vi "函数类型1测试 - 副本 (3).vi"() -> ()   [LabVIEW 2010]
panel:
  out "light_32":bool
  out "light_31":bool
  out "light_30":bool
  out "light_29":bool
  out "light_28":bool
  out "light_27":bool
  out "light_26":bool
  out "light_25":bool
  out "light_24":bool
  out "light_23":bool
  out "light_22":bool
  out "light_21":bool
  out "light_20":bool
  out "light_19":bool
  out "light_18":bool
  out "light_17":bool
  out "light_16":bool
  out "light_15":bool
  out "light_14":bool
  out "light_13":bool
  out "light_12":bool
  out "light_11":bool
  out "light_10":bool
  out "light_9":bool
  out "light_8":bool
  out "light_7":bool
  out "light_6":bool
  out "light_5":bool
  out "light_4":bool
  out "light_3":bool
  out "light_2":bool
  out "light_1":bool
  in  "A_16":bool
  in  "A_15":bool
  in  "A_14":bool
  in  "A_13":bool
  in  "A_12":bool
  in  "A_11":bool
  in  "A_10":bool
  in  "A_9":bool
  in  "A_8":bool
  in  "A_7":bool
  in  "A_6":bool
  in  "A_5":bool
  in  "A_4":bool
  in  "A_3":bool
  in  "A_2":bool
  in  "A_1":bool
  out "temp":string
  out "bstart":bool
  in  "同步_1":i32
  in  "数组_反馈值":dbl[][](array[numeric])
  in  "第几个数据":i32
  in  "第几组数据":i32
  out "Analog_WC":string[][](table) caption="表格"
  in  "数组_设定值":dbl[][](array[numeric])
  in  "数组_选择":bool[](array[boolean])
  out "Analog_back":string[][](table) caption="表格"
  in  "A_32":bool
  in  "A_31":bool
  in  "A_30":bool
  in  "A_29":bool
  in  "A_28":bool
  in  "A_27":bool
  in  "A_26":bool
  in  "A_25":bool
  in  "A_24":bool
  in  "A_23":bool
  in  "A_22":bool
  in  "A_21":bool
  in  "A_20":bool
  in  "A_19":bool
  in  "A_18":bool
  in  "A_17":bool
  in  "Analog_IN":string[][](table) caption="表格"
  out "退出？":bool
  out "合格？":bool[][](array[boolean])
  out "测试结论":string
  in  "btn_反选":bool
  in  "btn_全选":bool
  in  "btn_开始测试":bool
  in  "btn_取消":bool
  # "模拟量选择及输入值（V）"
  # "模拟量反馈值（V）"
  # "模拟量误差值（%）"
  # "从0开始"
  # "从1开始,第0列没有使用"
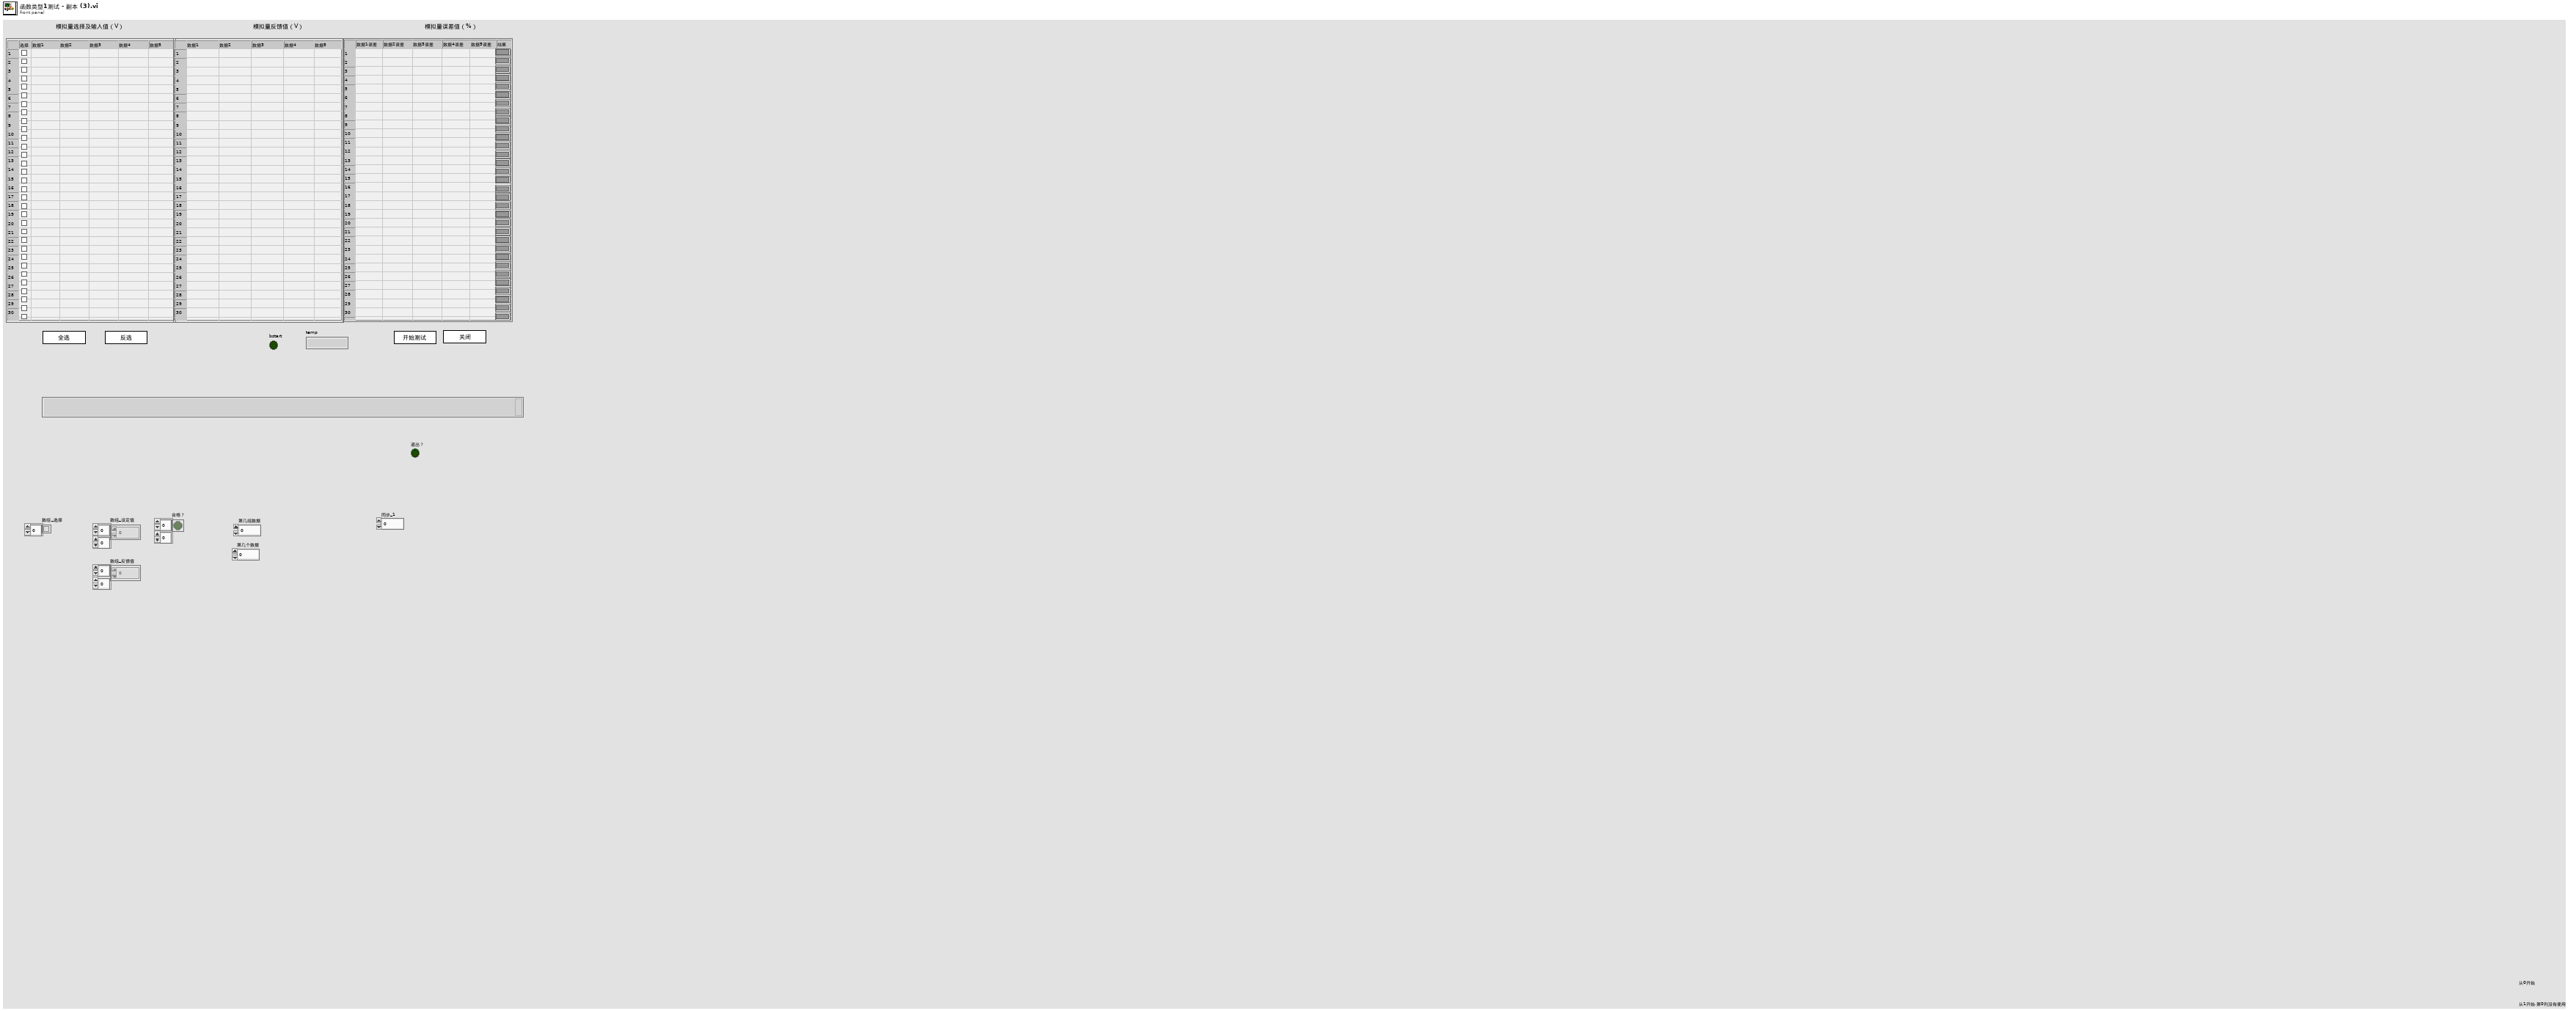
[diagram p1: front panel]
types:
  T1 = enum8{"Enabled", "Disabled", "Disabled and Grayed Out"}
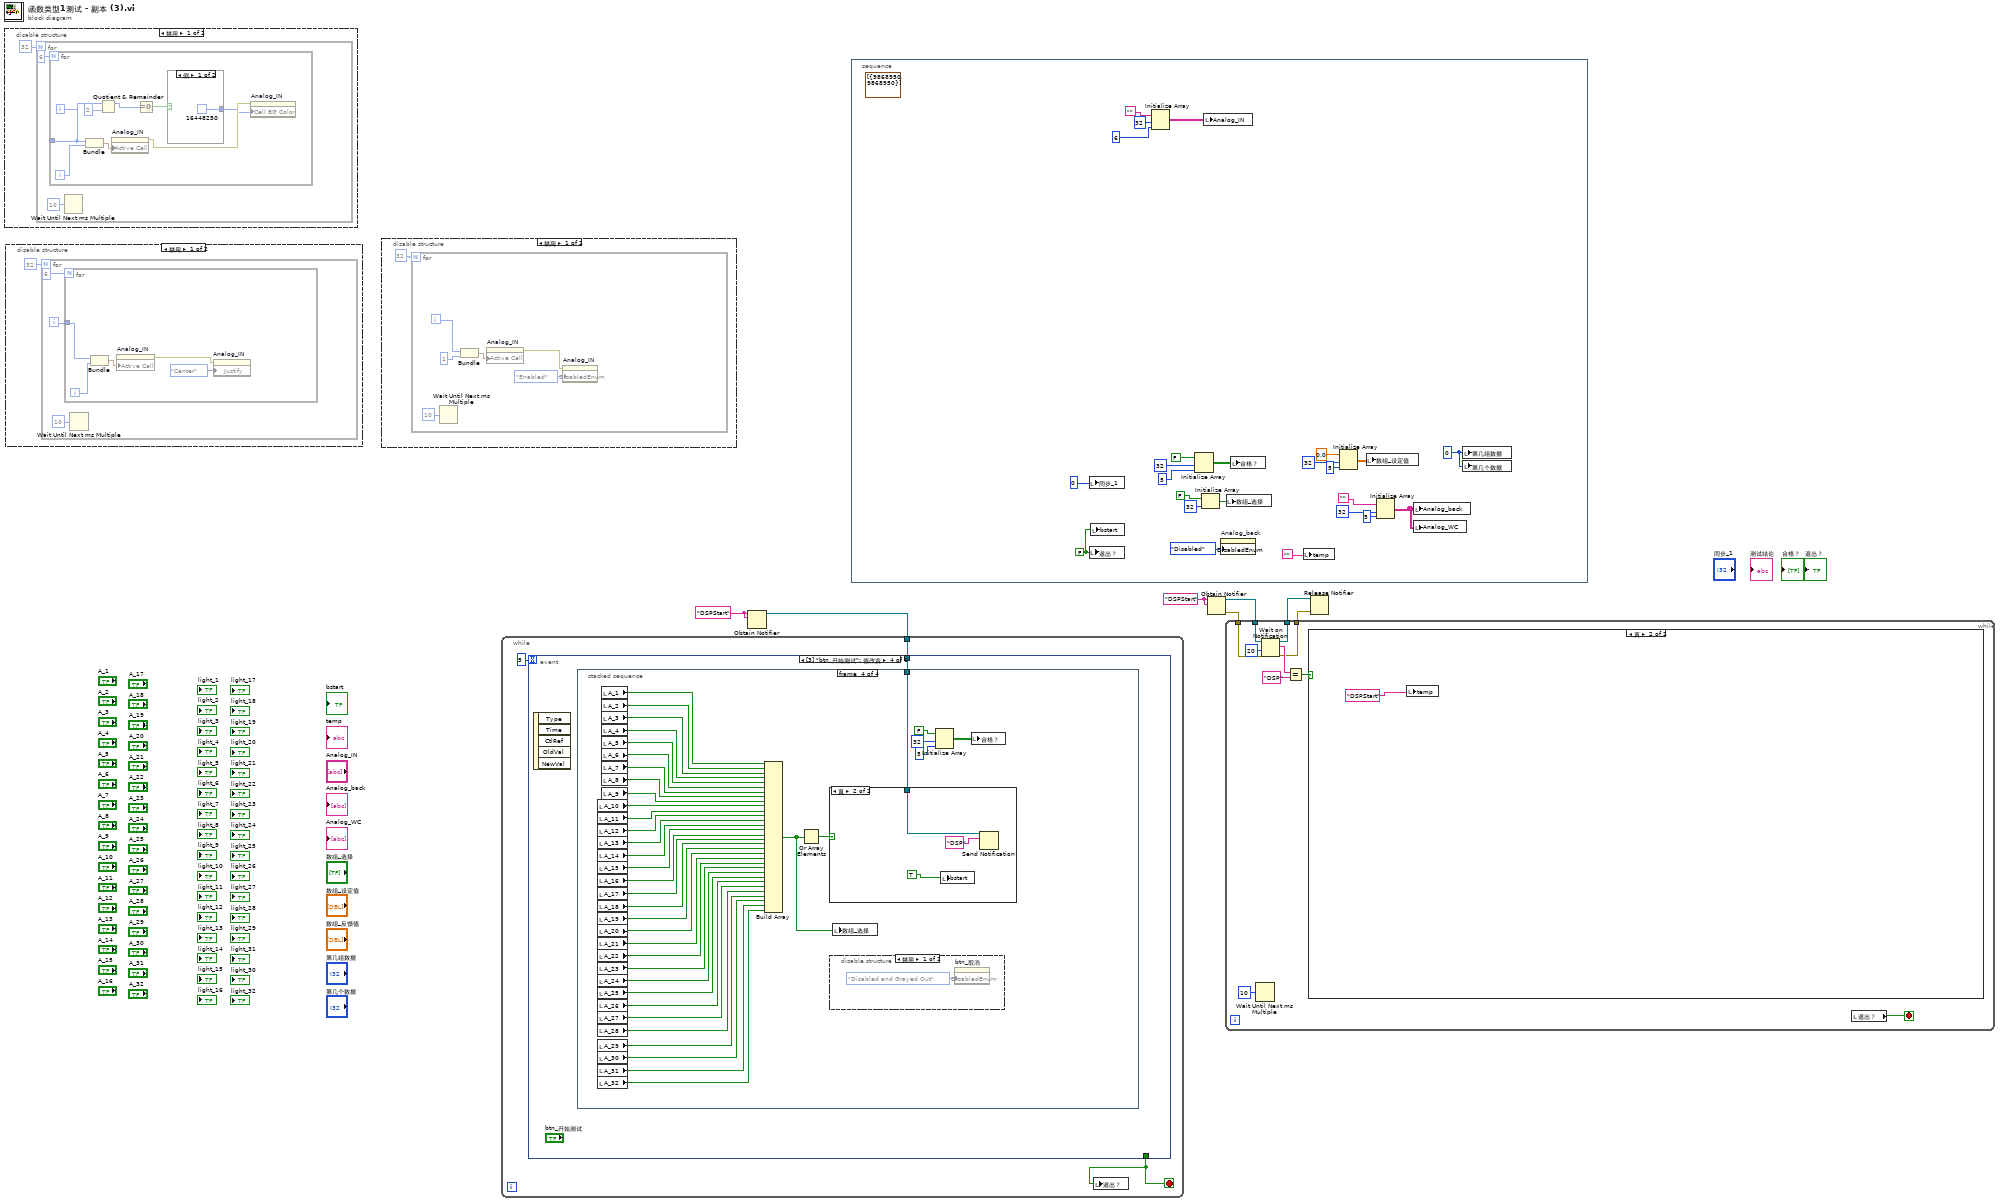
[diagram p0: block diagram]
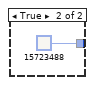
[diagram p2: hidden frame]
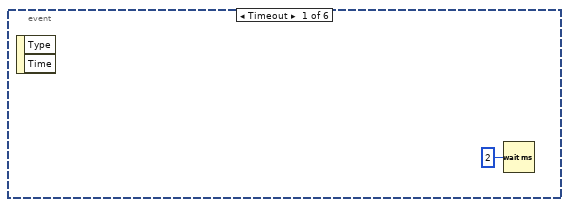
[diagram p7: hidden frame]
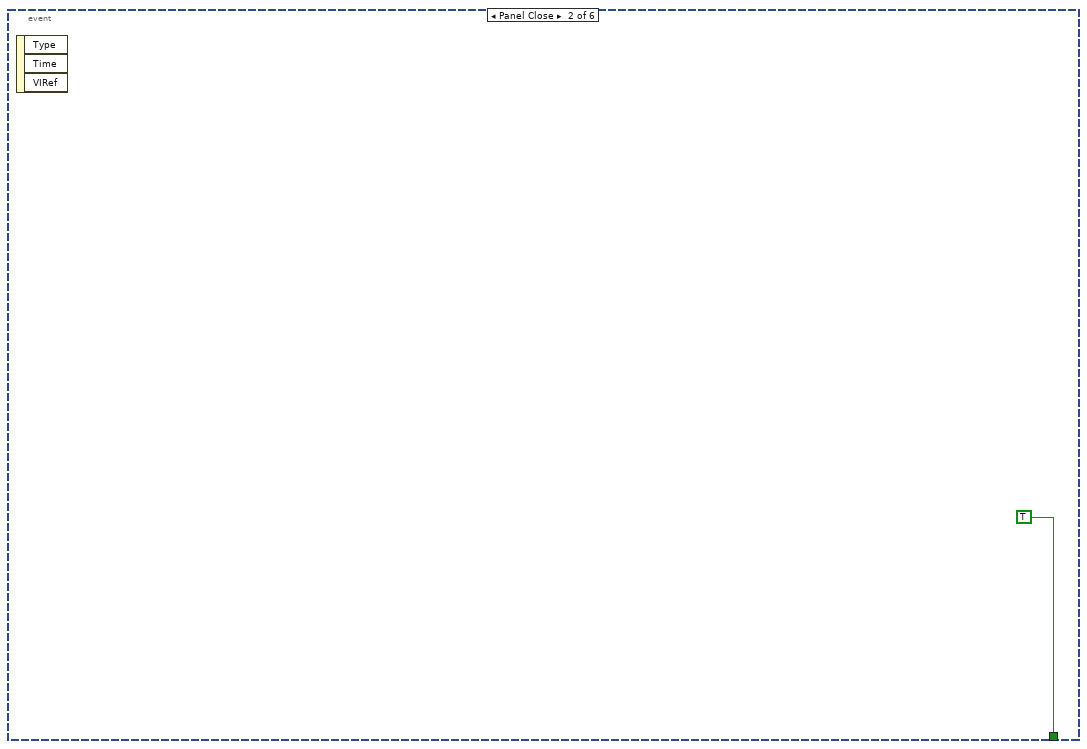
[diagram p8: hidden frame]
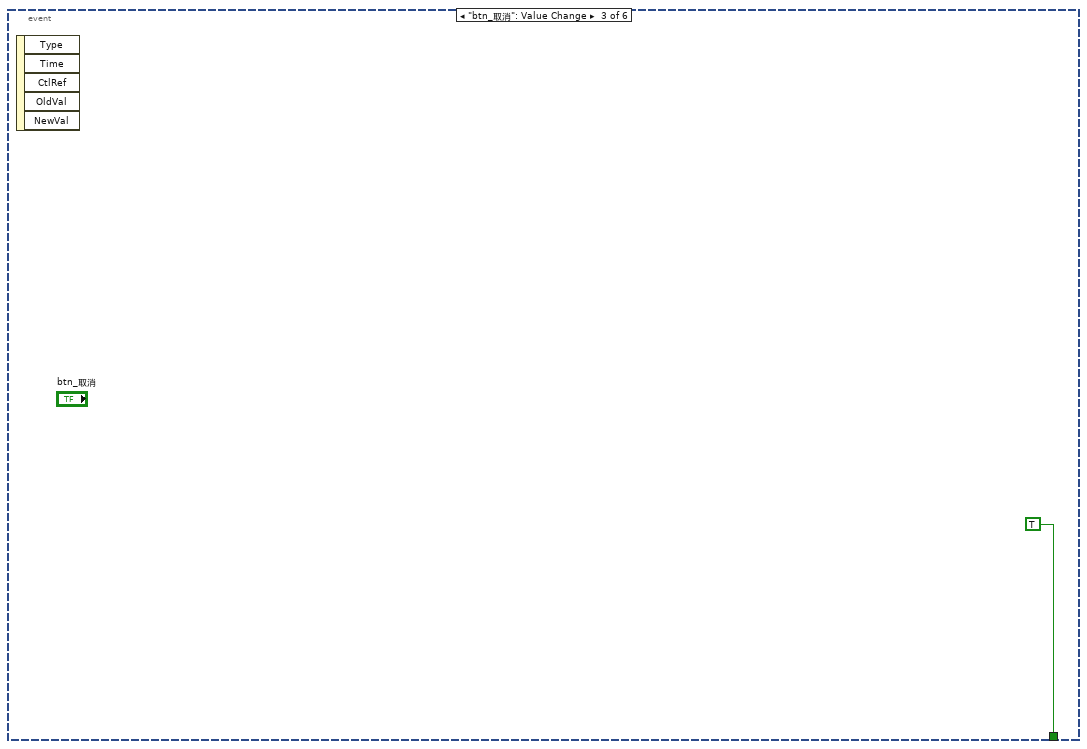
[diagram p9: hidden frame]
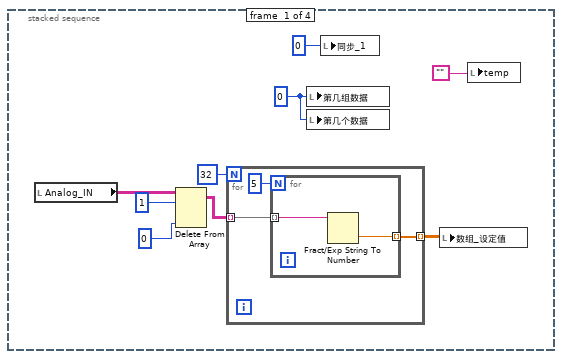
[diagram p10: hidden frame]
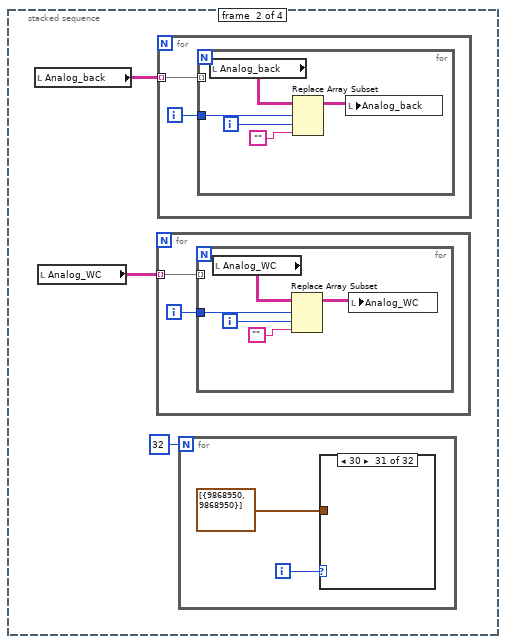
[diagram p11: hidden frame]
diagram:
  w2 = "DSPStart" ("名称（未命名）")
  w5 = "DSPStart" ("名称（未命名）")
  n1 = disable-structure shown="禁用" {
    frame Disabled {
      n2 = for {
        N: 32 -> [_]
        i -> [w10]
        n3 = for {
          N: 6 -> [_]
          tunnel: w10 -> [w18]
          i -> [w12]
          n4 = Bundle(w18, w12) -> (w15:cluster{i32, i32})  [unwired: 1 in]
          n5 = Quotient & Remainder(x=w18, y=2) -> (x-y*floor(x/y)=w16:i32)  [unwired: 1 out]
          n6 = property on="Analog_IN" class="Tbl (严格)"("Active Cell"=w15) -> (error out=w14:errorcluster)  [unwired: 2 in, 1 out]
          n7 = Equal To 0?(x=w16) -> (x = 0?=w19:bool)
          n8 = case shown="假" w19 {
            tunnel: [u32 16448250 u32 15723488] -> w13
            frame False {
            }
            frame True {
            }
          }
          n9 = property on="Analog_IN" class="Tbl (严格)"(error in=w14, "Cell BG Color"=w13) -> ()  [unwired: 1 in, 2 out]
        }
        n10 = Wait Until Next ms Multiple(millisecond multiple=u32 10 ("毫秒倍数")) -> ()  [unwired: 1 out]
      }
    }
    frame Enabled {
    }
  }
  n11 = disable-structure shown="禁用" {
    frame Disabled {
      n12 = for {
        N: 32 -> [_]
        i -> [w23]
        n13 = for {
          N: 6 -> [_]
          tunnel: w23 -> [w26]
          i -> [w27]
          n14 = Bundle(w26, w27) -> (w30:cluster{i32, i32})  [unwired: 1 in]
          n15 = property on="Analog_IN" class="Tbl (严格)"("Active Cell"=w30) -> (error out=w28:errorcluster)  [unwired: 2 in, 1 out]
          n16 = property on="Analog_IN" class="Tbl (严格)"(error in=w28, "Justify"=enum16{"Left", "Center", "Right"}."Center" ("活动单元格:单元格对齐")) -> ()  [unwired: 1 in, 2 out]
        }
        n17 = Wait Until Next ms Multiple(millisecond multiple=u32 10 ("毫秒倍数")) -> ()  [unwired: 1 out]
      }
    }
    frame Enabled {
    }
  }
  n18 = disable-structure shown="禁用" {
    frame Disabled {
      n19 = for {
        N: 32 -> [_]
        i -> [w36]
        n20 = Wait Until Next ms Multiple(millisecond multiple=u32 10 ("毫秒倍数")) -> ()  [unwired: 1 out]
        n21 = Bundle(w36, 1) -> (w35:cluster{i32, i32})  [unwired: 1 in]
        n22 = property on="Analog_IN" class="Tbl (严格)"("Active Cell"=w35) -> (error out=w32:errorcluster)  [unwired: 2 in, 1 out]
        n23 = property on="Analog_IN" class="Tbl (严格)"(error in=w32, "DisabledEnum"=T1."Enabled" ("禁用")) -> ()  [unwired: 1 in, 2 out]
      }
    }
    frame Enabled {
    }
  }
  n24 = Obtain Notifier(name (unnamed)=w2, notification data type=w2) -> (notifier out=w1:refnum<notifier>)  [unwired: 2 in, 2 out]
  n25 = while {
    tunnel: w1 -> [w39]
    stop <- w40 stop-if-true
    n26 = event shown="[3] \"btn_开始测试\": 值改变" {
      selector: _ -> [_ _ _ _ _ _]
      dyn-events: _ -> [_ _ _ _ _ _]
      timeout: 5 -> [_ _ _ _ _ _]
      tunnel: [_ TRUE TRUE _ _ _] -> w40
      tunnel: w39 -> [_ _ _ w44 _ _]
      event Timeout {
        n27 = event-data() -> ()  [unwired: 1 in, 2 out]
        n28 = Wait (ms)(milliseconds to wait=u32 2 ("等待时间（毫秒）")) -> ()  [unwired: 1 out]
      }
      event Panel Close {
        n29 = event-data() -> ()  [unwired: 1 in, 3 out]
      }
      event "btn_取消": Value Change {
        n30 = event-data() -> ()  [unwired: 1 in, 5 out]
      }
      event "btn_开始测试": Value Change {
        n31 = event-data() -> ()  [unwired: 1 in, 5 out]
        n32 = stacked-sequence {
          tunnel: w44 -> [_ _ _ w92]
          frame #0 {
            w46 = 0 ("第几组数据")
            n33 = local read "Analog_IN"() -> (w53:string[][])
            n34 = Delete From Array(array=w53, length=1 ("长度"), index (col)=0 ("禁用的索引 (列)")) -> (array with subset deleted=w49:string[][])  [unwired: 1 in, 1 out]
            n35 = for {
              N: 32 -> [_]
              tunnel: w49 -> [w56] mode=indexing
              tunnel: [w55] -> w52 mode=indexing
              n36 = for {
                N: 5 -> [_]
                tunnel: w56 -> [w58] mode=indexing
                tunnel: [w57] -> w55 mode=indexing
                n37 = Fract/Exp String To Number(string=w58) -> (number=w57:dbl)  [unwired: 3 in, 1 out]
              }
            }
            n38 = local write "第几组数据"(w46) -> ()
            n39 = local write "第几个数据"(w46) -> ()
            n40 = local write "同步_1"(0 ("同步_2")) -> ()
            n41 = local write "数组_设定值"(w52) -> ()
            n42 = local write "temp"("") -> ()
          }
          frame #1 {
            n43 = local read "Analog_back"() -> (w61:string[][])
            n44 = local read "Analog_WC"() -> (w60:string[][])
            n45 = for {
              tunnel: w60 -> [w65] mode=indexing
              i -> [w64]
              n46 = for {
                tunnel: w65 -> [_] mode=indexing
                tunnel: w64 -> [w69]
                i -> [w68]
                n47 = local read "Analog_WC"() -> (w70:string[][])
                n48 = Replace Array Subset(array=w70, new element="", index (row)=w69, index (col)=w68) -> (w66:string[][])
                n49 = local write "Analog_WC"(w66) -> ()
              }
            }
            n50 = for {
              tunnel: w61 -> [w72] mode=indexing
              i -> [w71]
              n51 = for {
                tunnel: w72 -> [_] mode=indexing
                tunnel: w71 -> [w76]
                i -> [w75]
                n52 = local read "Analog_back"() -> (w77:string[][])
                n53 = Replace Array Subset(array=w77, new element="", index (row)=w76, index (col)=w75) -> (w73:string[][])
                n54 = local write "Analog_back"(w73) -> ()
              }
            }
            n55 = for {
              N: 32 -> [_]
              i -> [w63]
              n56 = case shown="30" w63 {
                tunnel: cluster{u32, u32}[] [{9868950, 9868950}] -> [_ _ _ _ _ _ _ _ _ _ _ _ _ _ _ _ _ _ _ _ _ _ _ _ _ _ _ _ _ _ _ _]
                frame 0, Default {
                }
                frame 1 {
                }
                frame 2 {
                }
                frame 3 {
                }
                frame 4 {
                }
                frame 5 {
                }
                frame 6 {
                }
                frame 7 {
                }
                frame 8 {
                }
                frame 9 {
                }
                frame 10 {
                }
                frame 11 {
                }
                frame 12 {
                }
                frame 13 {
                }
                frame 14 {
                }
                frame 15 {
                }
                frame 16 {
                }
                frame 17 {
                }
                frame 18 {
                }
                frame 19 {
                }
                frame 20 {
                }
                frame 21 {
                }
                frame 22 {
                }
                frame 23 {
                }
                frame 24 {
                }
                frame 25 {
                }
                frame 26 {
                }
                frame 27 {
                }
                frame 28 {
                }
                frame 29 {
                }
                frame 30 {
                }
                frame 31 {
                }
              }
            }
          }
          frame #2 {
            n57 = for {
              N: 32 -> [_]
              i -> [w80]
              n58 = disable-structure shown="禁用" {
                frame Disabled {
                  n59 = Wait Until Next ms Multiple(millisecond multiple=u32 10 ("毫秒倍数")) -> ()  [unwired: 1 out]
                }
                frame Enabled {
                }
              }
              n60 = for {
                N: 6 -> [_]
                tunnel: w80 -> [w88]
                i -> [w85]
                n61 = Bundle(w88, w85) -> (w84:cluster{i32, i32})  [unwired: 1 in]
                n62 = Quotient & Remainder(x=w88, y=2) -> (x-y*floor(x/y)=w86:i32)  [unwired: 1 out]
                n63 = property on="Analog_WC" class="Tbl (严格)"("Active Cell"=w84) -> (error out=w83:errorcluster)  [unwired: 2 in, 1 out]
                n64 = Equal To 0?(x=w86) -> (x = 0?=w89:bool)
                n65 = case shown="假" w89 {
                  tunnel: [u32 16448250 u32 15723488] -> w82
                  frame False {
                  }
                  frame True {
                  }
                }
                n66 = property on="Analog_WC" class="Tbl (严格)"(error in=w83, "Cell BG Color"=w82) -> ()  [unwired: 1 in, 2 out]
              }
            }
          }
          frame #3 {
            n67 = local read "A_10"() -> (w121:bool)
            n68 = local read "A_11"() -> (w120:bool)
            n69 = local read "A_12"() -> (w119:bool)
            n70 = local read "A_13"() -> (w118:bool)
            n71 = local read "A_14"() -> (w117:bool)
            n72 = local read "A_15"() -> (w116:bool)
            n73 = local read "A_16"() -> (w115:bool)
            n74 = local read "A_17"() -> (w114:bool)
            n75 = local read "A_18"() -> (w113:bool)
            n76 = local read "A_19"() -> (w112:bool)
            n77 = local read "A_20"() -> (w111:bool)
            n78 = local read "A_21"() -> (w110:bool)
            n79 = local read "A_22"() -> (w109:bool)
            n80 = local read "A_23"() -> (w108:bool)
            n81 = local read "A_24"() -> (w107:bool)
            n82 = local read "A_25"() -> (w106:bool)
            n83 = local read "A_26"() -> (w105:bool)
            n84 = local read "A_27"() -> (w104:bool)
            n85 = local read "A_28"() -> (w103:bool)
            n86 = local read "A_29"() -> (w102:bool)
            n87 = local read "A_30"() -> (w101:bool)
            n88 = local read "A_31"() -> (w100:bool)
            n89 = local read "A_32"() -> (w99:bool)
            n90 = local read "A_1"() -> (w130:bool)
            n91 = local read "A_2"() -> (w129:bool)
            n92 = local read "A_3"() -> (w128:bool)
            n93 = local read "A_4"() -> (w127:bool)
            n94 = local read "A_5"() -> (w126:bool)
            n95 = local read "A_6"() -> (w125:bool)
            n96 = local read "A_7"() -> (w124:bool)
            n97 = local read "A_8"() -> (w123:bool)
            n98 = local read "A_9"() -> (w122:bool)
            n99 = Build Array(w130, w129, w128, w127, w126, w125, w124, w123, w122, w121, w120, w119, w118, w117, w116, w115, w114, w113, w112, w111, w110, w109, w108, w107, w106, w105, w104, w103, w102, w101, w100, w99) -> (w93:bool[])
            n100 = Or Array Elements(Boolean array=w93) -> (logical OR=w98:bool)
            n101 = disable-structure shown="禁用" {
              frame Disabled {
                n102 = property on="btn_取消" class="Bool"("DisabledEnum"=T1."Disabled and Grayed Out" ("禁用")) -> ()  [unwired: 2 in, 2 out]
              }
              frame Enabled {
              }
            }
            n103 = case shown="真" w98 {
              tunnel: w92 -> [_ w133]
              frame False {
                n104 = call "显示对话框信息"() -> ()  [unwired: 10 in, 2 out]
              }
              frame True {
                n105 = local write "bstart"(TRUE) -> ()
                n106 = Send Notification(notification="DSP" ("通知"), notifier=w133) -> ()  [unwired: 1 in, 2 out]
              }
            }
            n107 = local write "数组_选择"(w93) -> ()
            n108 = Initialize Array(FALSE, 32 ("维数大小"), 5 ("维数大小")) -> (w94:bool[][])
            n109 = local write "合格？"(w94) -> ()
          }
        }
      }
      event "btn_全选": Value Change {
        w135 = TRUE ("单选_AD_1")
        n110 = event-data() -> ()  [unwired: 1 in, 5 out]
        n111 = local write "A_1"(w135) -> ()
        n112 = local write "A_2"(w135) -> ()
        n113 = local write "A_3"(w135) -> ()
        n114 = local write "A_4"(w135) -> ()
        n115 = local write "A_5"(w135) -> ()
        n116 = local write "A_6"(w135) -> ()
        n117 = local write "A_7"(w135) -> ()
        n118 = local write "A_8"(w135) -> ()
        n119 = local write "A_9"(w135) -> ()
        n120 = local write "A_10"(w135) -> ()
        n121 = local write "A_11"(w135) -> ()
        n122 = local write "A_12"(w135) -> ()
        n123 = local write "A_13"(w135) -> ()
        n124 = local write "A_14"(w135) -> ()
        n125 = local write "A_15"(w135) -> ()
        n126 = local write "A_16"(w135) -> ()
        n127 = local write "A_17"(w135) -> ()
        n128 = local write "A_18"(w135) -> ()
        n129 = local write "A_19"(w135) -> ()
        n130 = local write "A_20"(w135) -> ()
        n131 = local write "A_21"(w135) -> ()
        n132 = local write "A_22"(w135) -> ()
        n133 = local write "A_23"(w135) -> ()
        n134 = local write "A_24"(w135) -> ()
        n135 = local write "A_25"(w135) -> ()
        n136 = local write "A_26"(w135) -> ()
        n137 = local write "A_27"(w135) -> ()
        n138 = local write "A_28"(w135) -> ()
        n139 = local write "A_29"(w135) -> ()
        n140 = local write "A_30"(w135) -> ()
        n141 = local write "A_31"(w135) -> ()
        n142 = local write "A_32"(w135) -> ()
      }
      event "btn_反选": Value Change {
        n143 = event-data() -> ()  [unwired: 1 in, 5 out]
        n144 = local read "A_17"() -> (w167:bool)
        n145 = local read "A_18"() -> (w165:bool)
        n146 = local read "A_19"() -> (w163:bool)
        n147 = local read "A_20"() -> (w161:bool)
        n148 = local read "A_21"() -> (w159:bool)
        n149 = local read "A_22"() -> (w157:bool)
        n150 = local read "A_23"() -> (w155:bool)
        n151 = local read "A_24"() -> (w153:bool)
        n152 = local read "A_25"() -> (w151:bool)
        n153 = local read "A_26"() -> (w149:bool)
        n154 = local read "A_27"() -> (w147:bool)
        n155 = local read "A_28"() -> (w145:bool)
        n156 = local read "A_29"() -> (w143:bool)
        n157 = local read "A_30"() -> (w141:bool)
        n158 = local read "A_31"() -> (w139:bool)
        n159 = local read "A_32"() -> (w137:bool)
        n160 = local read "A_1"() -> (w199:bool)
        n161 = local read "A_2"() -> (w197:bool)
        n162 = local read "A_3"() -> (w196:bool)
        n163 = local read "A_4"() -> (w195:bool)
        n164 = local read "A_5"() -> (w194:bool)
        n165 = local read "A_6"() -> (w193:bool)
        n166 = local read "A_7"() -> (w192:bool)
        n167 = local read "A_8"() -> (w191:bool)
        n168 = local read "A_9"() -> (w190:bool)
        n169 = local read "A_10"() -> (w189:bool)
        n170 = local read "A_11"() -> (w188:bool)
        n171 = local read "A_12"() -> (w187:bool)
        n172 = local read "A_13"() -> (w186:bool)
        n173 = local read "A_14"() -> (w185:bool)
        n174 = local read "A_15"() -> (w184:bool)
        n175 = local read "A_16"() -> (w183:bool)
        n176 = Not(x=w199) -> (.not. x?=w198:bool)
        n177 = Not(x=w197) -> (.not. x?=w168:bool)
        n178 = Not(x=w196) -> (.not. x?=w169:bool)
        n179 = Not(x=w195) -> (.not. x?=w170:bool)
        n180 = Not(x=w194) -> (.not. x?=w171:bool)
        n181 = Not(x=w193) -> (.not. x?=w172:bool)
        n182 = Not(x=w192) -> (.not. x?=w173:bool)
        n183 = Not(x=w191) -> (.not. x?=w174:bool)
        n184 = Not(x=w190) -> (.not. x?=w175:bool)
        n185 = Not(x=w189) -> (.not. x?=w176:bool)
        n186 = Not(x=w188) -> (.not. x?=w177:bool)
        n187 = Not(x=w187) -> (.not. x?=w178:bool)
        n188 = Not(x=w186) -> (.not. x?=w179:bool)
        n189 = Not(x=w185) -> (.not. x?=w180:bool)
        n190 = Not(x=w184) -> (.not. x?=w181:bool)
        n191 = Not(x=w183) -> (.not. x?=w182:bool)
        n192 = Not(x=w167) -> (.not. x?=w166:bool)
        n193 = Not(x=w165) -> (.not. x?=w164:bool)
        n194 = Not(x=w163) -> (.not. x?=w162:bool)
        n195 = Not(x=w161) -> (.not. x?=w160:bool)
        n196 = Not(x=w159) -> (.not. x?=w158:bool)
        n197 = Not(x=w157) -> (.not. x?=w156:bool)
        n198 = Not(x=w155) -> (.not. x?=w154:bool)
        n199 = Not(x=w153) -> (.not. x?=w152:bool)
        n200 = Not(x=w151) -> (.not. x?=w150:bool)
        n201 = Not(x=w149) -> (.not. x?=w148:bool)
        n202 = Not(x=w147) -> (.not. x?=w146:bool)
        n203 = Not(x=w145) -> (.not. x?=w144:bool)
        n204 = Not(x=w143) -> (.not. x?=w142:bool)
        n205 = Not(x=w141) -> (.not. x?=w140:bool)
        n206 = Not(x=w139) -> (.not. x?=w138:bool)
        n207 = Not(x=w137) -> (.not. x?=w136:bool)
        n208 = local write "A_1"(w198) -> ()
        n209 = local write "A_2"(w168) -> ()
        n210 = local write "A_3"(w169) -> ()
        n211 = local write "A_4"(w170) -> ()
        n212 = local write "A_5"(w171) -> ()
        n213 = local write "A_6"(w172) -> ()
        n214 = local write "A_7"(w173) -> ()
        n215 = local write "A_8"(w174) -> ()
        n216 = local write "A_9"(w175) -> ()
        n217 = local write "A_10"(w176) -> ()
        n218 = local write "A_11"(w177) -> ()
        n219 = local write "A_12"(w178) -> ()
        n220 = local write "A_13"(w179) -> ()
        n221 = local write "A_14"(w180) -> ()
        n222 = local write "A_15"(w181) -> ()
        n223 = local write "A_16"(w182) -> ()
        n224 = local write "A_17"(w166) -> ()
        n225 = local write "A_18"(w164) -> ()
        n226 = local write "A_19"(w162) -> ()
        n227 = local write "A_20"(w160) -> ()
        n228 = local write "A_21"(w158) -> ()
        n229 = local write "A_22"(w156) -> ()
        n230 = local write "A_23"(w154) -> ()
        n231 = local write "A_24"(w152) -> ()
        n232 = local write "A_25"(w150) -> ()
        n233 = local write "A_26"(w148) -> ()
        n234 = local write "A_27"(w146) -> ()
        n235 = local write "A_28"(w144) -> ()
        n236 = local write "A_29"(w142) -> ()
        n237 = local write "A_30"(w140) -> ()
        n238 = local write "A_31"(w138) -> ()
        n239 = local write "A_32"(w136) -> ()
      }
    }
    n240 = local write "退出？"(w40) -> ()
  }
  n241 = stacked-sequence {
    frame #0 {
      w206 = 0 ("第几组数据")
      w205 = FALSE ("退出？")
      (unwired) cluster{u32, u32}[] [{9868950, 9868950}]
      n242 = local write "同步_1"(0 ("同步_2")) -> ()
      n243 = local write "退出？"(w205) -> ()
      n244 = local write "bstart"(w205) -> ()
      n245 = Initialize Array("", 32 ("维数大小"), 6 ("维数大小")) -> (w203:string[][])
      n246 = Initialize Array(FALSE, 32 ("维数大小"), 5 ("维数大小")) -> (w220:bool[][])
      n247 = Initialize Array(FALSE, 32 ("维数大小")) -> (w210:bool[])
      n248 = local write "Analog_IN"(w203) -> ()
      n249 = property on="Analog_back" class="Tbl (严格)"("DisabledEnum"=T1."Disabled" ("禁用")) -> ()  [unwired: 2 in, 2 out]
      n250 = local write "数组_选择"(w210) -> ()
      n251 = local write "合格？"(w220) -> ()
      n252 = local write "temp"("") -> ()
      n253 = Initialize Array(0.0, 32 ("维数大小"), 5 ("维数大小")) -> (w213:dbl[][])
      n254 = local write "数组_设定值"(w213) -> ()
      n255 = Initialize Array("", 32 ("维数大小"), 5 ("维数大小")) -> (w217:string[][])
      n256 = local write "Analog_back"(w217) -> ()
      n257 = local write "Analog_WC"(w217) -> ()
      n258 = local write "第几组数据"(w206) -> ()
      n259 = local write "第几个数据"(w206) -> ()
    }
  }
  n260 = Obtain Notifier(name (unnamed)=w5, notification data type=w5) -> (notifier out=w7:refnum<notifier>, error out=w6:errorcluster)  [unwired: 2 in, 1 out]
  n261 = while {
    tunnel: w7 -> [w227]
    tunnel: w6 -> [w226]
    tunnel: [w225] -> w4
    tunnel: [w224] -> w3
    stop <- w229 stop-if-true
    n262 = Wait Until Next ms Multiple(millisecond multiple=u32 10 ("毫秒倍数")) -> ()  [unwired: 1 out]
    n263 = Wait on Notification(notifier=w227, timeout in ms (-1)=20 ("超时毫秒(-1)"), error in (no error)=w226) -> (notifier out=w225:refnum<notifier>, notification=w233:string, error out=w224:errorcluster)  [unwired: 1 in, 1 out]
    n264 = Equal?(x=w233, y="DSP" ("通知")) -> (x = y?=w230:bool)
    n265 = case shown="真" w230 {
      frame False {
      }
      frame True {
        n266 = local write "temp"("DSPStart" ("名称（未命名）")) -> ()
      }
    }
    n267 = local read "退出？"() -> (w229:bool)
  }
  n268 = Release Notifier(notifier=w4, error in (no error)=w3) -> ()  [unwired: 1 in, 3 out]
